vi "RT - Main.vi"() -> ()   [LabVIEW 2016]
uses:
  Target SubVIs/Notes.ctl
  <vilib>/FPGAPlugInAG/myRIO-1900/niLvFpga_Open_myRIO-1900.vi
  <vilib>/rvi/interface/common/dynamic/niFpgaDynamicAddResources.vi
  <vilib>/FPGAPlugInAG/Dynamic/niLvFpga_Run_Dynamic.vi
  <vilib>/Utility/error.llb/Error Cluster From Error Code.vi
  <vilib>/rvi/errors/niLvFpgaAdjustHostInterfaceError.vi
  <vilib>/rvi/interface/nirviOpenFPGA/nirviOpenFPGA.xnode
  FPGA Bitfiles/myRIOMusicBox_FPGATarget_FPGATopLevel_2nGkaHAX2zM.lvbitx
  FPGA Files/FPGA Top Level.vi
  <vilib>/rvi/interface/nirviMethod/nirviMethod.xnode
  <vilib>/rvi/interface/nirviReadWriteControl/nirviReadWriteControl.xnode
  <vilib>/rvi/interface/Simulation/niFpgaSimulationCallBeginRW.vi
  NiFpgaLv.dll
panel:
  in  "x":u32=50
  out "Event Number":i32
  out "Note Events":T1[](array[typedef])
  in  "Stop Sending":bool
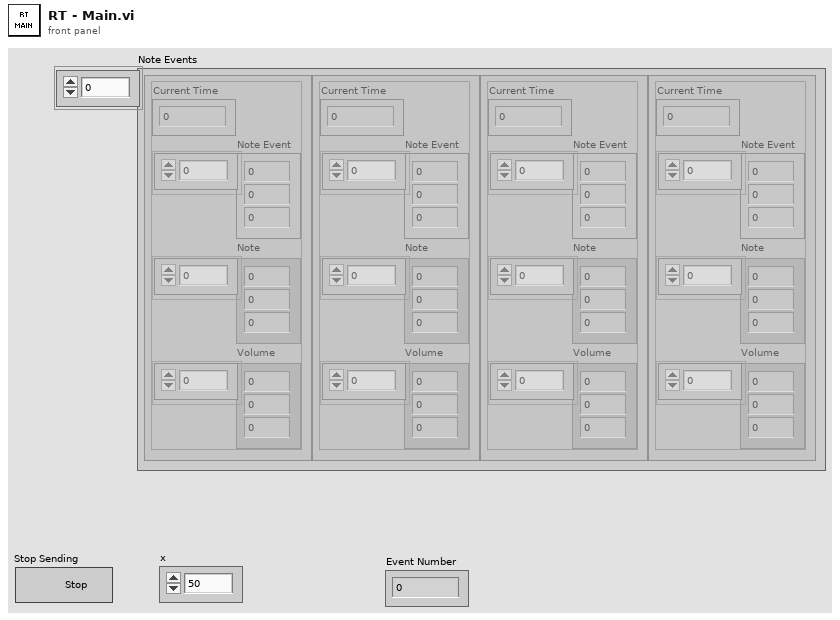
[diagram p1: front panel]
types:
  T1 = typedef "Notes.ctl" = cluster{"Current Time":u32, "Note Event":u32[], "Note":u32[], "Volume":u32[]}
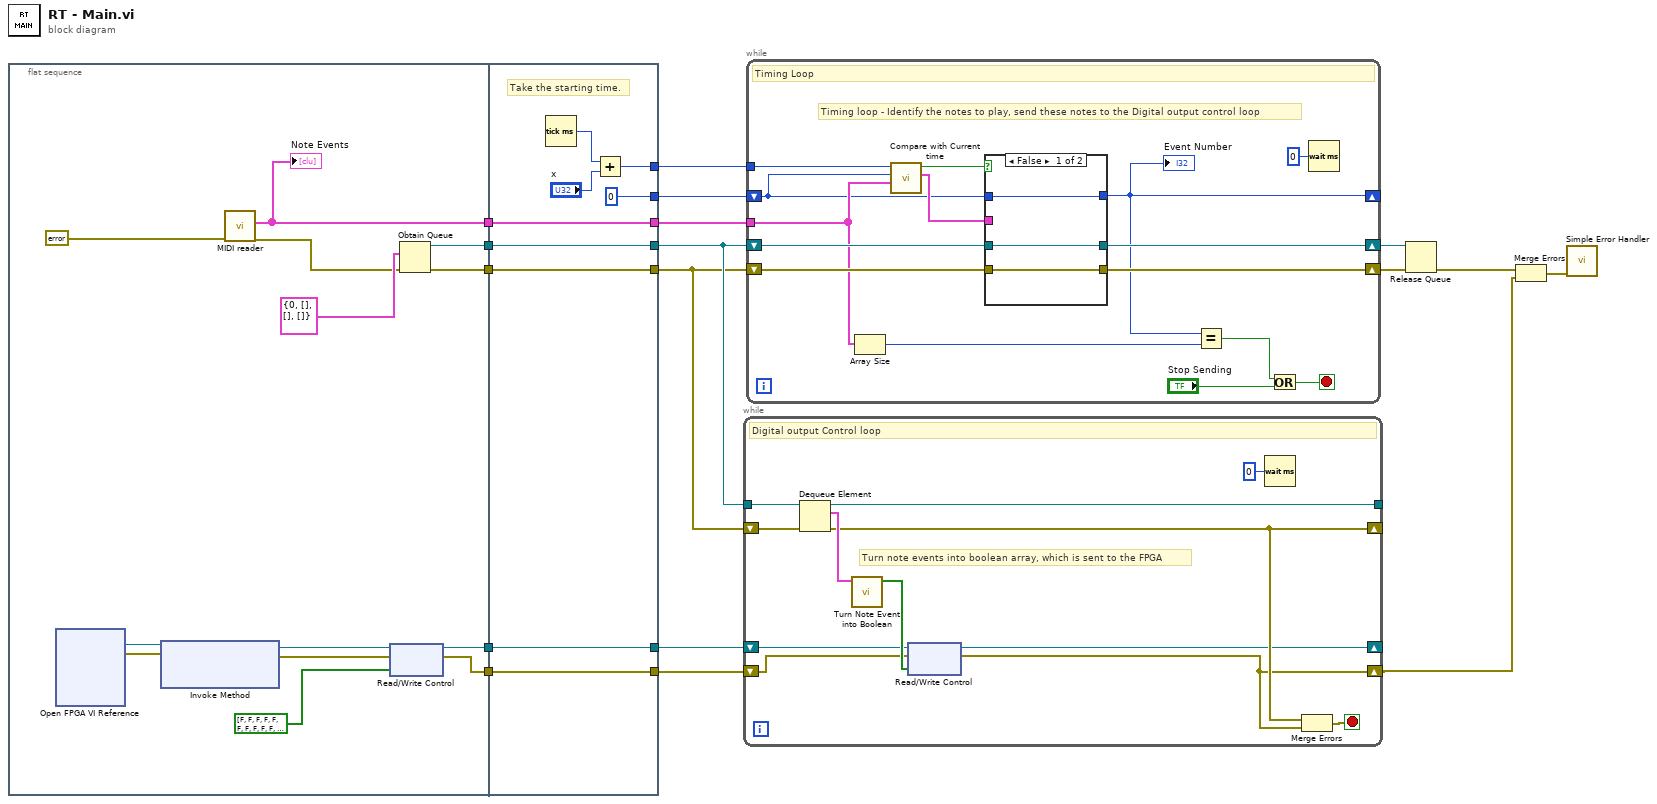
[diagram p0: block diagram]
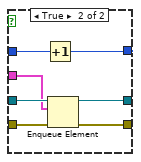
[diagram p2: hidden frame]
diagram:
  n1 = flat-sequence {
    tunnel: [w19] -> w17
    tunnel: [w30] -> w16
    tunnel: [w29] -> w15
    tunnel: [w27] -> w14
    tunnel: [w26] -> w13
    tunnel: [w35] -> w5
    tunnel: [w36] -> w6
    tunnel: [w37] -> w10
    tunnel: [w38] -> w11
    tunnel: [w39] -> w12
    tunnel: w17 -> [w39]
    tunnel: w16 -> [w38]
    tunnel: w15 -> [w37]
    tunnel: w14 -> [w36]
    tunnel: w13 -> [w35]
    tunnel: [w32] -> w3
    tunnel: [0] -> w2
    frame #0 {
      n2 = xnode "Open FPGA VI Reference"() -> ("FPGA VI Reference Out"=w22:refnum<k20>, "error out"=w21:errorcluster)  [unwired: 2 in]
      n3 = xnode "Invoke Method"("FPGA VI Reference In"=w22, "error in"=w21) -> ("FPGA VI Reference Out"=w25:refnum<k20>, "error out"=w24:errorcluster)  [unwired: 1 in]
      n4 = call "MIDI reader.vi"("error in"=errorcluster {"status"=FALSE, "code"=0, "source"=""}) -> ("error out"=w20:errorcluster, "Note Events"=w19:T1[])  [unwired: 8 in, 1 out]
      "Note Events" <- w19
      n5 = xnode "Read/Write Control"("FPGA VI Reference In"=w25, "error in"=w24, "Array"=bool[] [FALSE, FALSE, FALSE, FALSE, FALSE, FALSE, FALSE, FALSE, FALSE, FALSE, FALSE, FALSE]) -> ("FPGA VI Reference Out"=w26:refnum<k20>, "error out"=w27:errorcluster)
      n6 = Obtain Queue(element data type=T1 {"Current Time"=0, "Note Event"=[], "Note"=[], "Volume"=[]} ("element"), error in (no error)=w20) -> (queue out=w30:refnum<queue>, error out=w29:errorcluster)  [unwired: 3 in, 1 out]
    }
    frame #1 {
      # "Take the starting time."
      n7 = Tick Count (ms)() -> (millisecond timer value=w33:u32)
      n8 = Add(x=w33, y="x") -> (x+y=w32:u32)
    }
  }
  n9 = while {
    shift-right: [w46] -> _
    shift-left: w10 -> [w50]
    shift-right: [w44] -> w1
    shift-left: w6 -> [w40]
    tunnel: w11 -> [w51]
    tunnel: [w49] -> _
    shift-right: [w43] -> _
    shift-left: w5 -> [w41]
    stop <- w42 stop-if-true
    # "Turn note events into boolean array, which is sent to the FPGA"
    # "Digital output Control loop"
    n10 = Dequeue Element(queue=w51, error in (no error)=w50) -> (queue out=w49:refnum<queue>, element=w47:T1, error out=w46:errorcluster)  [unwired: 1 in, 1 out]
    n11 = call "Turn Note Event into Boolean.vi"("element"=w47) -> ("Boolean array"=w45:bool[])  [unwired: 10 in]
    n12 = xnode "Read/Write Control"("FPGA VI Reference In"=w41, "error in"=w40, "Array"=w45) -> ("FPGA VI Reference Out"=w43:refnum<k20>, "error out"=w44:errorcluster)
    n13 = Wait (ms)(milliseconds to wait=u32 0) -> ()  [unwired: 1 out]
    n14 = Merge Errors(w46, w44) -> (w42:errorcluster)
  }
  n15 = while {
    tunnel: w3 -> [w53]
    tunnel: w12 -> [w55]
    shift-right: [w57] -> _
    shift-left: w2 -> [w54]
    shift-right: [w62] -> w8
    shift-left: w10 -> [w64]
    shift-right: [w63] -> w9
    shift-left: w11 -> [w65]
    stop <- w60 stop-if-true
    # "Timing loop - Identify the notes to play, send these notes to the Digital output control loop"
    # "Timing Loop"
    n16 = Array Size(array=w55) -> (size(s)=w59:i32)
    n17 = call "Compare with Current time.vi"("Note Events"=w55, "Numeric Control 2"=w54, "Numeric Control"=w53) -> ("Array"=w56:T1, "Boolean"=w52:bool)  [unwired: 7 in]
    n18 = case shown="False" w52 {
      tunnel: [w69 w71] -> w57
      tunnel: w54 -> [w69 w76]
      tunnel: w65 -> [w68 w75]
      tunnel: w64 -> [w67 w74]
      tunnel: w56 -> [_ w70]
      tunnel: [w68 w73] -> w63
      tunnel: [w67 w72] -> w62
      frame False {
      }
      frame True {
        n19 = Increment(x=w76) -> (x+1=w71:i32)
        n20 = Enqueue Element(queue=w75, element=w70, error in (no error)=w74) -> (queue out=w73:refnum<queue>, error out=w72:errorcluster)  [unwired: 1 in, 1 out]
      }
    }
    "Event Number" <- w57
    n21 = Equal?(x=w57, y=w59) -> (x = y?=w58:bool)
    n22 = Or(x=w58, y="Stop Sending") -> (x .or. y?=w60:bool)
    n23 = Wait (ms)(milliseconds to wait=u32 0) -> ()  [unwired: 1 out]
  }
  n24 = Release Queue(queue=w9, error in (no error)=w8) -> (error out=w7:errorcluster)  [unwired: 1 in, 2 out]
  n25 = Merge Errors(w7, w1) -> (w4:errorcluster)
  n26 = call <vilib>:"Simple Error Handler.vi"("error in (no error)"=w4) -> ()  [unwired: 4 in, 5 out]
